vi "WebDAV transfer.vi"(0 "IPstring":string, 2 "Mode":enum16{"Setup", "Retrieve File", "Export File"}(ring), 7 "Local Folder":path, 9 "Filename":string, 11 "Error In":errorcluster) -> (15 "Error Out":errorcluster)   [LabVIEW 2019]
uses:
  <vilib>/WebDAVClient/Advanced/Put File.vi
  <vilib>/WebDAVClient/Advanced/Get File.vi
  <vilib>/WebDAVClient/NI_WebDAV.lvlib
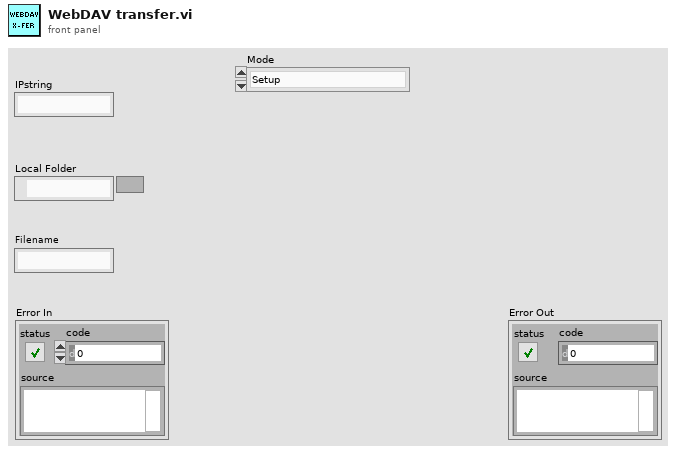
[diagram p1: front panel]
types:
  T1 = typedef "NI_WebDAV.lvlib/SessionHandle.ctl" = refnum<k1>
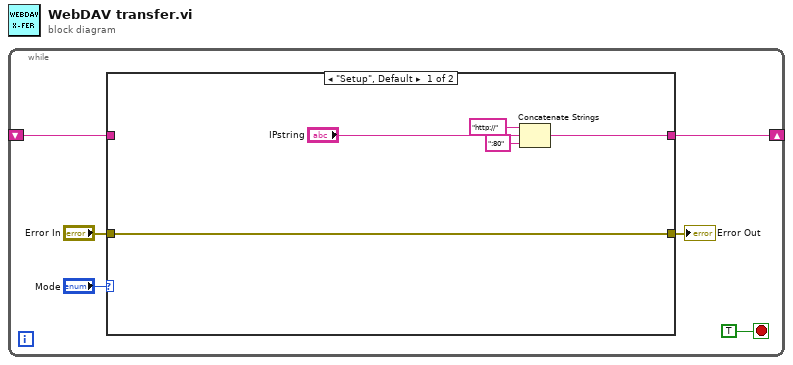
[diagram p0: block diagram]
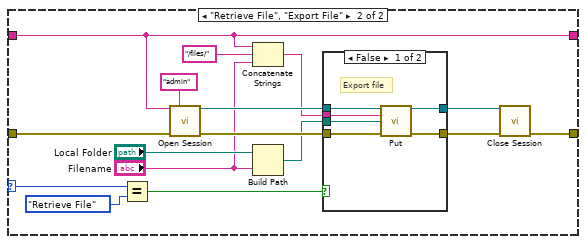
[diagram p2: hidden frame]
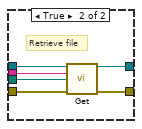
[diagram p3: hidden frame]
diagram:
  n1 = while {
    shift-right: [w4] -> _
    shift-left: _ -> [w3]
    stop <- TRUE stop-if-true
    n2 = case shown="\"Setup\", Default" "Mode" {
      selector: "Mode" -> [_ w25]
      tunnel: [w8 w18] -> w4
      tunnel: w3 -> [_ w18]
      tunnel: [w7 w13] -> w2
      tunnel: "Error In" -> [w7 w12]
      frame "Setup", Default {
        n3 = Concatenate Strings("http://" ("string"), "IPstring", ":80" ("string")) -> (w8:string)
      }
      frame "Retrieve File", "Export File" {
        n4 = Equal?(x=w25, y=enum16{"Setup", "Retrieve File", "Export File"}."Retrieve File" ("Mode")) -> (x = y?=w23:bool)
        n5 = call <vilib>:"Open Session.vi"("host uri prefix"=w18, "username"="admin", "error in (no error)"=w12) -> ("session handle out"=w22:T1, "error out"=w21:errorcluster)  [unwired: 11 in]
        n6 = Concatenate Strings(w18, "/files/" ("string"), "Filename") -> (w17:string)
        n7 = Build Path(base path="Local Folder", name or relative path="Filename") -> (appended path=w14:path)
        n8 = case shown="False" w23 {
          tunnel: w22 -> [w33 w39]
          tunnel: w21 -> [w32 w38]
          tunnel: [w31 w37] -> w20
          tunnel: [w30 w36] -> w19
          tunnel: w17 -> [w29 w35]
          tunnel: w14 -> [w28 w34]
          frame False {
            # "Export file"
            n9 = call-poly <vilib>:"Put.vi"("session handle"=w33, "relative uri"=w29, "local file path"=w28, "error in (no error)"=w32) -> ("session handle out"=w31:T1, "error out"=w30:errorcluster)  [unwired: 9 in, 1 out]
          }
          frame True {
            # "Retrieve file"
            n10 = call-poly <vilib>:"Get.vi"("session handle"=w39, "relative uri"=w35, "local file path"=w34, "error in (no error)"=w38) -> ("session handle out"=w37:T1, "error out"=w36:errorcluster)  [unwired: 9 in, 1 out]
          }
        }
        n11 = call <vilib>:"Close Session.vi"("session handle"=w20, "error in (no error)"=w19) -> ("error out"=w13:errorcluster)  [unwired: 13 in]
      }
    }
    "Error Out" <- w2
  }
